vi "Remote Client.vi"(6 "timeout (ms) [500]":i32=500, 8 "error in (no error)":errorcluster, 9 "Data in":variant, 10 "Command in":variant, 11 "Instrument in":refnum<class "Instrument.lvclass">) -> (0 "error out":errorcluster, 1 "Data out":variant, 2 "Command out":string, 3 "Instrument out":refnum<class "Instrument.lvclass">)   [LabVIEW 2019, in "Instrument.lvlib" / "Instrument.lvclass"]
doc: "Send a message to a remote Instrument process. This VI automatically handles checking support for requested command, Open, Send (Request), Receive (Response), Parses Responses, and finally closes the connection.\n\n<b>Command in</b> can be an Enum or String\n\n<b>Data in</b> is a Variant containing your data payload. The transport layer will format this data how it wishes (e.f. RemoteControl.ZMQ will create a JSON-RPC request object)\n\n<b>Data out</b> will adapt to <b>Data out type</b>.\n\nNote: if you need to send and receive high speed messages this is not the VI for you...you are better off using <b>Local Client.vi</b> or Instrument.sendMessageToProcess.vi</b>, both of which will give you better control over how data is flattened (or not)."
uses:
  Instrument.lvclass
panel:
  # "Remote Client.vi"
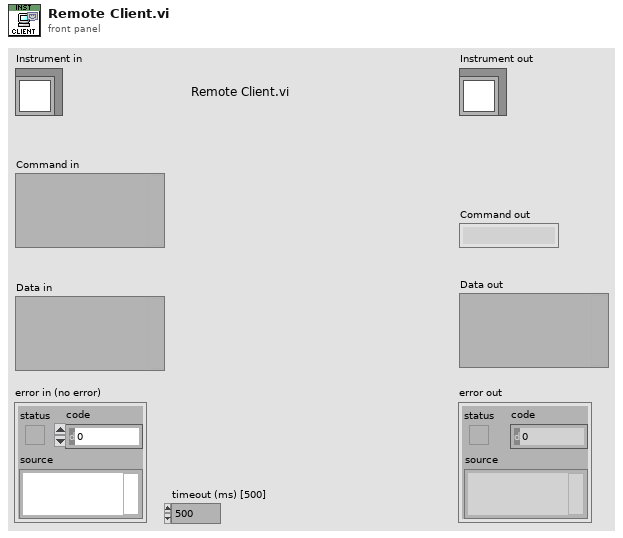
[diagram p1: front panel]
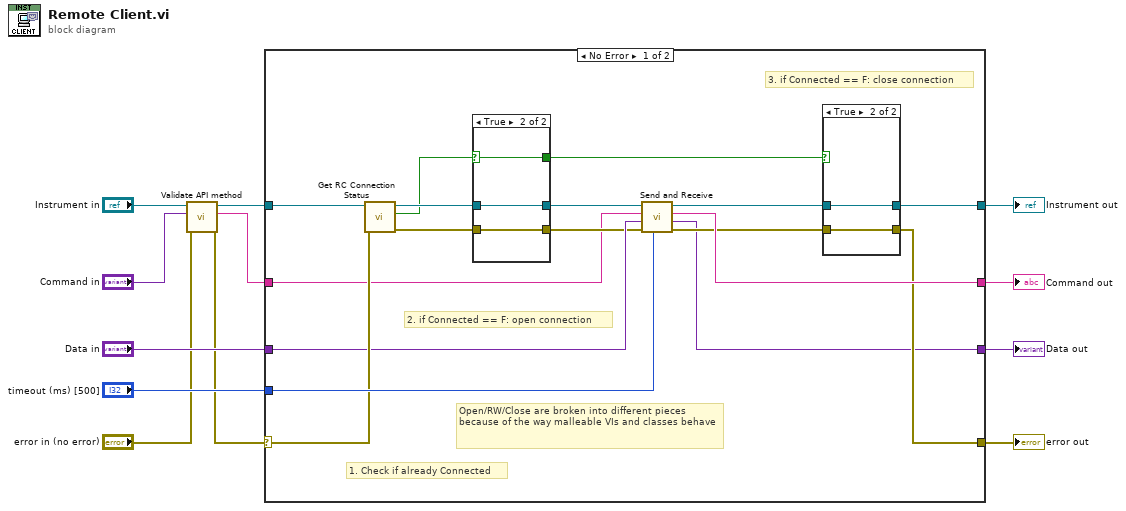
[diagram p0: block diagram]
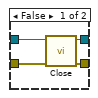
[diagram p2: hidden frame]
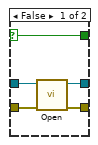
[diagram p3: hidden frame]
diagram:
  n1 = call "Validate API method.vi"("error in (no error)"="error in (no error)", "Command in"="Command in", "Instrument in"="Instrument in") -> ("error out"=w3:errorcluster, "command out"=w5:string, "Instrument out"=w1:refnum<class "Instrument.lvclass">)  [unwired: 6 in]
  n2 = case shown="No Error" w3 {
    selector: w3 -> [w25 w45]
    tunnel: [w14 w45] -> w12
    tunnel: [w29 w44] -> w11
    tunnel: w1 -> [w26 w44]
    tunnel: [w13 _] -> w10
    tunnel: [w27 _] -> w9
    tunnel: w5 -> [w17 _]
    tunnel: "Data in" -> [w19 _]
    tunnel: "timeout (ms) [500]" -> [w28 _]
    frame No Error {
      # "Open/RW/Close are broken into different pieces because of the way malleable VIs and classes behave"
      # "3. if Connected == F: close connection"
      # "2. if Connected == F: open connection"
      # "1. Check if already Connected"
      n3 = call "Get RC Connection Status.vi"("error in (no error)"=w25, "Instrument in"=w26) -> ("error out"=w21:errorcluster, "RC Connected?"=w20:bool, "Instrument out"=w22:refnum<class "Instrument.lvclass">)  [unwired: 7 in]
      n4 = case shown="True" w20 {
        selector: w20 -> [w36 w41]
        tunnel: [w40 w42] -> w24
        tunnel: [w39 w43] -> w18
        tunnel: w22 -> [w38 w42]
        tunnel: w21 -> [w37 w43]
        tunnel: [w36 w41] -> w16
        frame False {
          n5 = call-dynamic "Open.vi"("error in (no error)"=w37, "Instrument in"=w38) -> ("error out"=w39:errorcluster, "Instrument out"=w40:refnum<class "Instrument.lvclass">)  [unwired: 8 in]
        }
        frame True {
        }
      }
      n6 = call "Send and Receive.vi"("timeout (ms) [500]"=w28, "error in (no error)"=w18, "Data in"=w19, "Command in"=w17, "Instrument in"=w24) -> ("error out"=w15:errorcluster, "Data out"=w13:variant, "Command out"=w27:string, "Instrument out"=w23:refnum<class "Instrument.lvclass">)  [unwired: 3 in]
      n7 = case shown="True" w16 {
        tunnel: w23 -> [w33 w35]
        tunnel: [w32 w35] -> w29
        tunnel: [w31 w34] -> w14
        tunnel: w15 -> [w30 w34]
        frame False {
          n8 = call-dynamic "Close.vi"("error in (no error)"=w30, "Instrument in"=w33) -> ("error out"=w31:errorcluster, "Instrument out"=w32:refnum<class "Instrument.lvclass">)  [unwired: 8 in]
        }
        frame True {
        }
      }
    }
    frame Error {
    }
  }
  "error out" <- w12
  "Instrument out" <- w11
  "Command out" <- w9
  "Data out" <- w10
